vi "E816_All_VIs.vi"   [LabVIEW 2020]
doc: "This VI contains all high level and low level VIs valid for E-816. \nSee diagram for a survey of all E-816 high level and low level VIs. \nMenu / Browse / Show VI Hierarchy will show the file paths of the VIs. \nGlobal Variables are shown as Control as well as Indicator."
uses:
  Low Level/Communication.llb/Global1.vi
  Low Level/General command.llb/Controller names.ctl
  Low Level/Support.llb/Unbunde/bundle interface clusters for PI Terminal.vi
  Low Level/Communication.llb/Available DLL interfaces.ctl
  Low Level/Communication.llb/Available DLLs.ctl
  Low Level/Communication.llb/Available interfaces.ctl
  Low Level/Communication.llb/Termination character.ctl
  Low Level/General command.llb/Global2 (Array).vi
  Low Level/Communication.llb/Global DaisyChain.vi
  Low Level/Analog control.llb/Available Analog Commands.ctl
  Low Level/Analog control.llb/Global Analog.vi
panel:
  # "E-816 PI GCS LabVIEW driver set"
  # "This VI contains all high level and low level VIs valid for E-816. See diagram for a survey of all E-816 high \nlevel and low level VIs. Menu / Browse / Show VI Hierarchy will show the file paths of the VIs. Global \nVariables are shown as Control as well as Indicator."
types:
  T1 = typedef "Available Analog Commands.ctl" = enum16{"INITIALIZE", "VOL?", "VOL ", "CLOSE", "MOV", "POS?", "VCO", "VCO?", "WAIT_WF", "TMN?", "TMX?", "VEL", "VEL?", "SAI?", "MVR", "ERR?", "#24", "STP", "*IDN?", "#5", "STE", "DRR?", "W_Wave", "HLP?", "W/R_Wave"}
  T2 = typedef "Termination character.ctl" = enum16{"LF", "CR", "LFCR", "CRLF"}
  T3 = typedef "Available interfaces.ctl" = u16
  T4 = typedef "Available DLLs.ctl" = u16
  T5 = typedef "Available DLL interfaces.ctl" = u16
  T6 = typedef "Controller names.ctl" = enum16{"None", "Analog", "C-702", "C-843", "C-843.PM", "C-844", "C-848", "C-865", "C-866", "C-867", "C-880", "E-516", "E-517", "E-709", "E-710", "E-712", "E-725", "E-753", "E-755", "E-761", "E-816", "E-861", "F-206", "M-840", "M-850", "M-8X0", "Mercury", "Mercury_GCS"}
  T7 = cluster{"Conversion factor":dbl[], "Velocity":dbl[], "Velocity control mode":bool, "AO.Resolution":dbl, "Lower voltage limit (V)":dbl, "Upper voltage limit (V)":dbl, "AO_WF_T (s)":dbl, "AI Sample Rate":dbl, "AI Samples/Channel":i32, "Hyperbit":bool, "Offset (V)":dbl[], "Hyperbit StayOnPos":bool, "Gain (V)":dbl[], "Bit rate (Hz)":dbl, "PWM rate (Hz)":dbl, "HyperBit Password":string, "AO.MaxRate":dbl, "Conversion offset":dbl[]}[]
  T8 = cluster{"No. of devices":i32, "Port ID":i32, "Devices":string[], "Description":string}[]
  T9 = cluster{"Conn. axes":string[], "Controller name":T6}[]
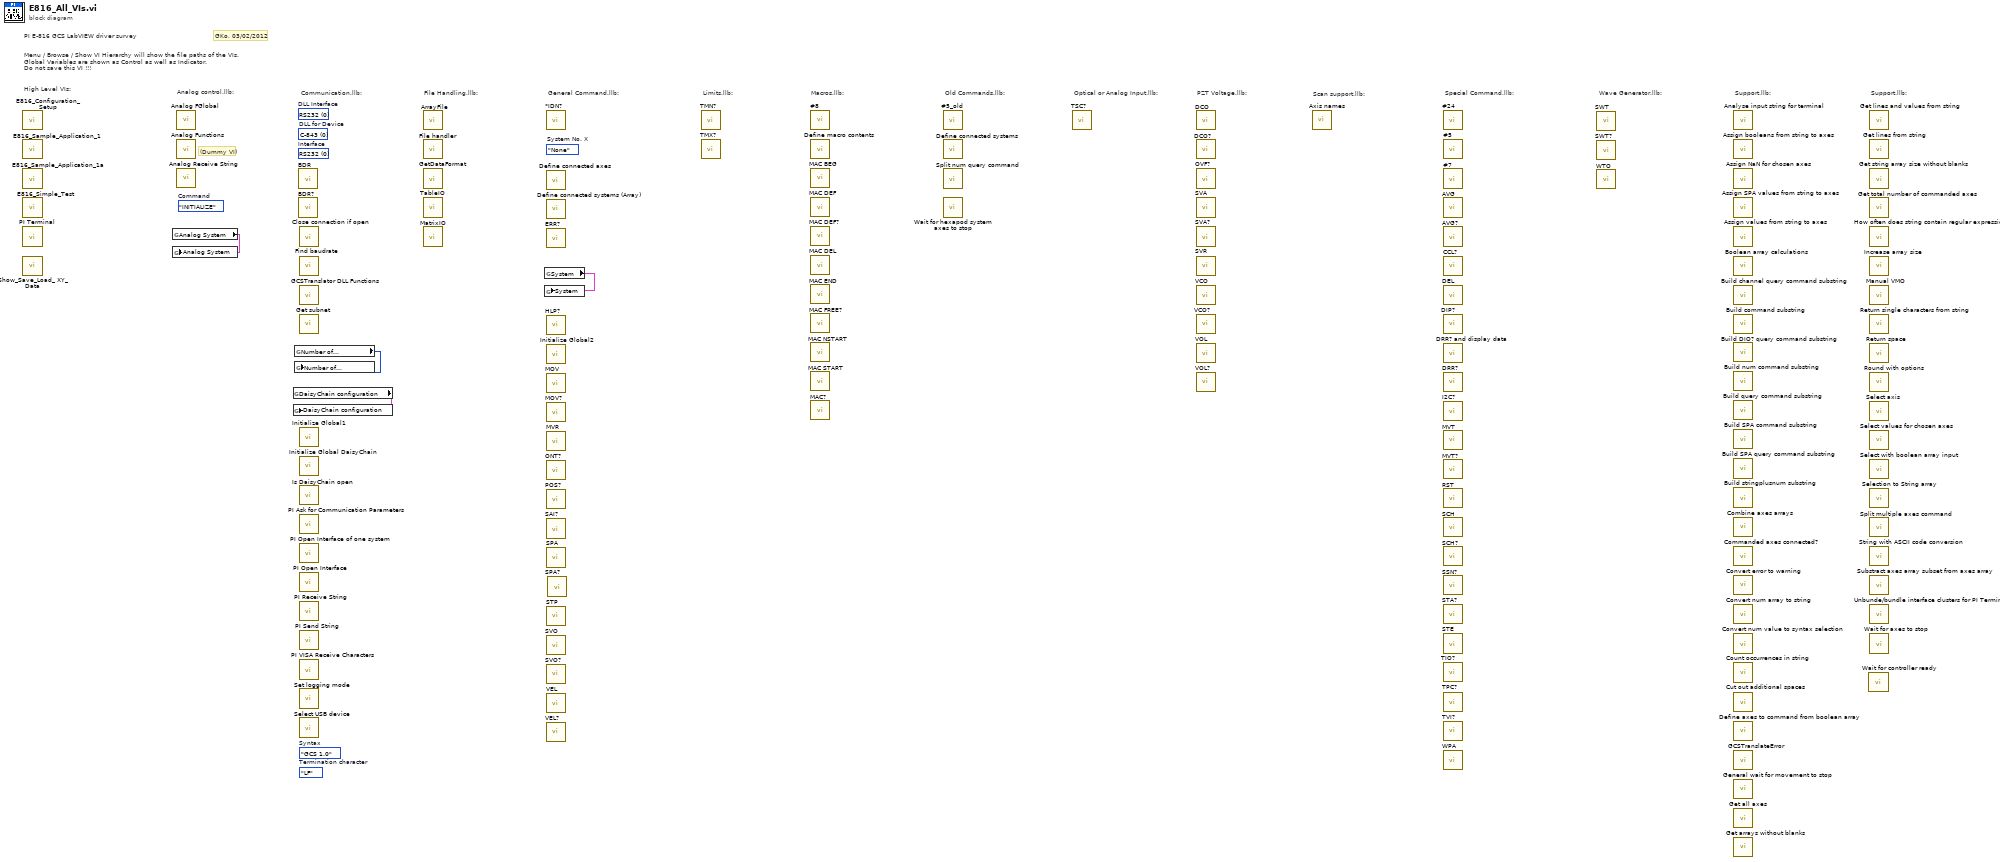
[diagram p0: block diagram]
diagram:
  (unwired) Available_Analog_Commands."INITIALIZE"  # Command
  (unwired) Termination_character."LF"  # Termination character
  (unwired) enum16{"GCS 1.0", "GCS 2.0"}."GCS 1.0"  # Syntax
  (unwired) T3 0 items=["RS232", "GPIB", "DLL", "TCP-IP"]  # Interface
  (unwired) T4 0 items=["C-843", "C-844", "E-710", "C-843.PM", "C-865", "E-761", "Mercury"]  # DLL for Device
  (unwired) T5 0 items=["RS232", "GPIB", "Board", "TCP-IP", "USB"]  # DLL Interface
  (unwired) Controller_names."None"  # System No. X
  # "Macros.llb:"
  # "Scan support.llb:"
  # "(Dummy VI)"
  # "GKo, 03/02/2012"
  # "High Level VIs:"
  # "Analog control.llb:"
  # "Support.llb:"
  # "Wave Generator.llb:"
  # "Support.llb:"
  # "Special Command.llb:"
  # "PZT Voltage.llb:"
  # "Optical or Analog Input.llb:"
  # "Old Commands.llb:"
  # "Limits.llb:"
  # "General Command.llb:"
  # "File Handling.llb:"
  # "Menu / Browse / Show VI Hierarchy will show the file paths of the VIs. \nGlobal Variables are shown as Control as well as Indicator.\nDo not save this VI !!!"
  # "PI E-816 GCS LabVIEW driver survey"
  # "Communication.llb:"
  n1 = call "E816_Configuration_Setup.vi"() -> ()  [unwired: 10 in, 10 out]
  n2 = call "E816_Sample_Application_1.vi"() -> ()  [unwired: 20 out]
  n3 = call "E816_Sample_Application_1a.vi"() -> ()  [unwired: 20 out]
  n4 = call "E816_Simple_Test.vi"() -> ()  [unwired: 20 out]
  n5 = call "PI Terminal.vi"() -> ()  [unwired: 20 out]
  n6 = call "Show_Save_Load_ XY_Data.vi"() -> ()  [unwired: 7 in, 13 out]
  n7 = global read "Global Analog.vi" "Analog System"() -> (w1:T7)
  n8 = global write "Global Analog.vi" "Analog System"(w1) -> ()
  n9 = call "Analog FGlobal.vi"() -> ()  [unwired: 3 in, 17 out]
  n10 = call "Analog Functions.vi"() -> ()  [unwired: 7 in, 13 out]
  n11 = call "Analog Receive String.vi"() -> ()  [unwired: 5 in, 15 out]
  n12 = global read "Global DaisyChain.vi" "DaisyChain configuration"() -> (w2:T8)
  n13 = global write "Global DaisyChain.vi" "DaisyChain configuration"(w2) -> ()
  n14 = global read "Global1.vi" "Number of\nsystems"() -> (w4:i32)
  n15 = global write "Global1.vi" "Number of\nsystems"(w4) -> ()
  n16 = call "BDR.vi"() -> ()  [unwired: 4 in, 16 out]
  n17 = call "BDR?.vi"() -> ()  [unwired: 2 in, 18 out]
  n18 = call "Close connection if open.vi"() -> ()  [unwired: 3 in, 17 out]
  n19 = call "Find baudrate.vi"() -> ()  [unwired: 10 in, 10 out]
  n20 = call "GCSTranslator DLL Functions.vi"() -> ()  [unwired: 7 in, 13 out]
  n21 = call "Get subnet.vi"() -> ()  [unwired: 20 out]
  n22 = call "Initialize Global1.vi"() -> ()  [unwired: 2 in, 18 out]
  n23 = call "Initialize Global DaisyChain.vi"() -> ()  [unwired: 2 in, 18 out]
  n24 = call "Is DaisyChain open.vi"() -> ()  [unwired: 2 in, 18 out]
  n25 = call "PI Ask for Communication Parameters.vi"() -> ()  [unwired: 20 out]
  n26 = call "PI Open Interface of one system.vi"() -> ()  [unwired: 12 in, 8 out]
  n27 = call "PI Open Interface.vi"() -> ()  [unwired: 12 in, 8 out]
  n28 = call "PI Receive String.vi"() -> ()  [unwired: 3 in, 17 out]
  n29 = call "PI Send String.vi"() -> ()  [unwired: 4 in, 16 out]
  n30 = call "PI VISA Receive Characters.vi"() -> ()  [unwired: 3 in, 17 out]
  n31 = call "Set logging mode.vi"() -> ()  [unwired: 4 in, 16 out]
  n32 = call "Select USB device.vi"() -> ()  [unwired: 5 in, 15 out]
  n33 = call "ArrayFile.vi"() -> ()  [unwired: 20 out]
  n34 = call "File handler.vi"() -> ()  [unwired: 6 in, 14 out]
  n35 = call "GetDataFormat.vi"() -> ()  [unwired: 2 in, 18 out]
  n36 = call "TableIO.vi"() -> ()  [unwired: 6 in, 14 out]
  n37 = call "MatrixIO.vi"() -> ()  [unwired: 7 in, 13 out]
  n38 = global read "Global2 (Array).vi" "System"() -> (w3:T9)
  n39 = global write "Global2 (Array).vi" "System"(w3) -> ()
  n40 = call "*IDN?.vi"() -> ()  [unwired: 2 in, 18 out]
  n41 = call "Define connected axes.vi"() -> ()  [unwired: 5 in, 15 out]
  n42 = call "Define connected systems (Array).vi"() -> ()  [unwired: 4 in, 16 out]
  n43 = call "ERR?.vi"() -> ()  [unwired: 2 in, 18 out]
  n44 = call "HLP?.vi"() -> ()  [unwired: 2 in, 18 out]
  n45 = call "Initialize Global2.vi"() -> ()  [unwired: 2 in, 18 out]
  n46 = call "MOV.vi"() -> ()  [unwired: 5 in, 15 out]
  n47 = call "MOV?.vi"() -> ()  [unwired: 5 in, 15 out]
  n48 = call "MVR.vi"() -> ()  [unwired: 5 in, 15 out]
  n49 = call "ONT?.vi"() -> ()  [unwired: 5 in, 15 out]
  n50 = call "POS?.vi"() -> ()  [unwired: 5 in, 15 out]
  n51 = call "SAI?.vi"() -> ()  [unwired: 5 in, 15 out]
  n52 = call "SPA.vi"() -> ()  [unwired: 10 in, 10 out]
  n53 = call "STP.vi"() -> ()  [unwired: 5 in, 15 out]
  n54 = call "SVO.vi"() -> ()  [unwired: 5 in, 15 out]
  n55 = call "SVO?.vi"() -> ()  [unwired: 5 in, 15 out]
  n56 = call "VEL.vi"() -> ()  [unwired: 6 in, 14 out]
  n57 = call "VEL?.vi"() -> ()  [unwired: 5 in, 15 out]
  n58 = call "SPA?.vi"() -> ()  [unwired: 7 in, 13 out]
  n59 = call "TMN?.vi"() -> ()  [unwired: 5 in, 15 out]
  n60 = call "TMX?.vi"() -> ()  [unwired: 5 in, 15 out]
  n61 = call "#8.vi"() -> ()  [unwired: 2 in, 18 out]
  n62 = call "Define macro contents.vi"() -> ()  [unwired: 3 in, 17 out]
  n63 = call "MAC BEG.vi"() -> ()  [unwired: 3 in, 17 out]
  n64 = call "MAC DEF.vi"() -> ()  [unwired: 3 in, 17 out]
  n65 = call "MAC DEF?.vi"() -> ()  [unwired: 2 in, 18 out]
  n66 = call "MAC DEL.vi"() -> ()  [unwired: 4 in, 16 out]
  n67 = call "MAC END.vi"() -> ()  [unwired: 2 in, 18 out]
  n68 = call "MAC FREE?.vi"() -> ()  [unwired: 2 in, 18 out]
  n69 = call "MAC NSTART.vi"() -> ()  [unwired: 5 in, 15 out]
  n70 = call "MAC START.vi"() -> ()  [unwired: 4 in, 16 out]
  n71 = call "MAC?.vi"() -> ()  [unwired: 4 in, 16 out]
  n72 = call "#5_old.vi"() -> ()  [unwired: 2 in, 18 out]
  n73 = call "Define connected systems.vi"() -> ()  [unwired: 4 in, 16 out]
  n74 = call "Split num query command.vi"() -> ()  [unwired: 4 in, 16 out]
  n75 = call "Wait for hexapod system axes to stop.vi"() -> ()  [unwired: 5 in, 15 out]
  n76 = call "TSC?.vi"() -> ()  [unwired: 2 in, 18 out]
  n77 = call "DCO.vi"() -> ()  [unwired: 4 in, 16 out]
  n78 = call "DCO?.vi"() -> ()  [unwired: 5 in, 15 out]
  n79 = call "OVF?.vi"() -> ()  [unwired: 5 in, 15 out]
  n80 = call "SVA.vi"() -> ()  [unwired: 5 in, 15 out]
  n81 = call "SVA?.vi"() -> ()  [unwired: 5 in, 15 out]
  n82 = call "SVR.vi"() -> ()  [unwired: 5 in, 15 out]
  n83 = call "VCO.vi"() -> ()  [unwired: 4 in, 16 out]
  n84 = call "VCO?.vi"() -> ()  [unwired: 5 in, 15 out]
  n85 = call "VOL.vi"() -> ()  [unwired: 5 in, 15 out]
  n86 = call "VOL?.vi"() -> ()  [unwired: 5 in, 15 out]
  n87 = call "Axis names.vi"() -> ()  [unwired: 1 in, 19 out]
  n88 = call "#24.vi"() -> ()  [unwired: 2 in, 18 out]
  n89 = call "#5.vi"() -> ()  [unwired: 2 in, 18 out]
  n90 = call "#7.vi"() -> ()  [unwired: 2 in, 18 out]
  n91 = call "AVG.vi"() -> ()  [unwired: 3 in, 17 out]
  n92 = call "AVG?.vi"() -> ()  [unwired: 2 in, 18 out]
  n93 = call "CCL?.vi"() -> ()  [unwired: 2 in, 18 out]
  n94 = call "DEL.vi"() -> ()  [unwired: 3 in, 17 out]
  n95 = call "DIP?.vi"() -> ()  [unwired: 5 in, 15 out]
  n96 = call "DRR? and display data.vi"() -> ()  [unwired: 7 in, 13 out]
  n97 = call "DRR?.vi"() -> ()  [unwired: 7 in, 13 out]
  n98 = call "I2C?.vi"() -> ()  [unwired: 2 in, 18 out]
  n99 = call "MVT.vi"() -> ()  [unwired: 5 in, 15 out]
  n100 = call "MVT?.vi"() -> ()  [unwired: 5 in, 15 out]
  n101 = call "RST.vi"() -> ()  [unwired: 5 in, 15 out]
  n102 = call "SCH.vi"() -> ()  [unwired: 3 in, 17 out]
  n103 = call "SCH?.vi"() -> ()  [unwired: 2 in, 18 out]
  n104 = call "SSN?.vi"() -> ()  [unwired: 4 in, 16 out]
  n105 = call "STA?.vi"() -> ()  [unwired: 5 in, 15 out]
  n106 = call "STE.vi"() -> ()  [unwired: 6 in, 14 out]
  n107 = call "TIO?.vi"() -> ()  [unwired: 2 in, 18 out]
  n108 = call "TPC?.vi"() -> ()  [unwired: 2 in, 18 out]
  n109 = call "TVI?.vi"() -> ()  [unwired: 3 in, 17 out]
  n110 = call "WPA.vi"() -> ()  [unwired: 7 in, 13 out]
  n111 = call "SWT.vi"() -> ()  [unwired: 6 in, 14 out]
  n112 = call "SWT?.vi"() -> ()  [unwired: 4 in, 16 out]
  n113 = call "WTO.vi"() -> ()  [unwired: 6 in, 14 out]
  n114 = call "Analyse input string for terminal.vi"() -> ()  [unwired: 2 in, 18 out]
  n115 = call "Assign booleans from string to axes.vi"() -> ()  [unwired: 5 in, 15 out]
  n116 = call "Assign NaN for chosen axes.vi"() -> ()  [unwired: 4 in, 16 out]
  n117 = call "Assign SPA values from string to axes.vi"() -> ()  [unwired: 7 in, 13 out]
  n118 = call "Assign values from string to axes.vi"() -> ()  [unwired: 6 in, 14 out]
  n119 = call "Boolean array calculations.vi"() -> ()  [unwired: 4 in, 16 out]
  n120 = call "Build channel query command substring.vi"() -> ()  [unwired: 7 in, 13 out]
  n121 = call "Build command substring.vi"() -> ()  [unwired: 7 in, 13 out]
  n122 = call "Build DIO? query command substring.vi"() -> ()  [unwired: 6 in, 14 out]
  n123 = call "Build num command substring.vi"() -> ()  [unwired: 3 in, 17 out]
  n124 = call "Build query command substring.vi"() -> ()  [unwired: 5 in, 15 out]
  n125 = call "Build SPA command substring.vi"() -> ()  [unwired: 10 in, 10 out]
  n126 = call "Build SPA query command substring.vi"() -> ()  [unwired: 5 in, 15 out]
  n127 = call "Build stringplusnum substring.vi"() -> ()  [unwired: 10 in, 10 out]
  n128 = call "Combine axes arrays.vi"() -> ()  [unwired: 2 in, 18 out]
  n129 = call "Commanded axes connected?.vi"() -> ()  [unwired: 3 in, 17 out]
  n130 = call "Convert error to warning.vi"() -> ()  [unwired: 2 in, 18 out]
  n131 = call "Convert num array to string.vi"() -> ()  [unwired: 2 in, 18 out]
  n132 = call "Convert num value to syntax selection.vi"() -> ()  [unwired: 1 in, 19 out]
  n133 = call "Count occurrences in string.vi"() -> ()  [unwired: 2 in, 18 out]
  n134 = call "Cut out additional spaces.vi"() -> ()  [unwired: 2 in, 18 out]
  n135 = call "Define axes to command from boolean array.vi"() -> ()  [unwired: 4 in, 16 out]
  n136 = call "GCSTranslateError.vi"() -> ()  [unwired: 1 in, 19 out]
  n137 = call "General wait for movement to stop.vi"() -> ()  [unwired: 8 in, 12 out]
  n138 = call "Get all axes.vi"() -> ()  [unwired: 1 in, 19 out]
  n139 = call "Get arrays without blanks.vi"() -> ()  [unwired: 3 in, 17 out]
  n140 = call "Wait for controller ready.vi"() -> ()  [unwired: 4 in, 16 out]
  n141 = call "Get lines and values from string.vi"() -> ()  [unwired: 2 in, 18 out]
  n142 = call "Get lines from string.vi"() -> ()  [unwired: 3 in, 17 out]
  n143 = call "Get string array size without blanks.vi"() -> ()  [unwired: 1 in, 19 out]
  n144 = call "Get total number of commanded axes.vi"() -> ()  [unwired: 2 in, 18 out]
  n145 = call "How often does string contain regular expression?.vi"() -> ()  [unwired: 2 in, 18 out]
  n146 = call "Increase array size.vi"() -> ()  [unwired: 3 in, 17 out]
  n147 = call "Manual VMO.vi"() -> ()  [unwired: 6 in, 14 out]
  n148 = call "Return single characters from string.vi"() -> ()  [unwired: 3 in, 17 out]
  n149 = call "Return space.vi"() -> ()  [unwired: 2 in, 18 out]
  n150 = call "Round with options.vi"() -> ()  [unwired: 4 in, 16 out]
  n151 = call "Select axis.vi"() -> ()  [unwired: 2 in, 18 out]
  n152 = call "Select values for chosen axes.vi"() -> ()  [unwired: 5 in, 15 out]
  n153 = call "Select with boolean array input.vi"() -> ()  [unwired: 4 in, 16 out]
  n154 = call "Selection to String array.vi"() -> ()  [unwired: 2 in, 18 out]
  n155 = call "Split multiple axes command.vi"() -> ()  [unwired: 9 in, 11 out]
  n156 = call "String with ASCII code conversion.vi"() -> ()  [unwired: 1 in, 19 out]
  n157 = call "Substract axes array subset from axes array.vi"() -> ()  [unwired: 2 in, 18 out]
  n158 = call "Unbunde/bundle interface clusters for PI Terminal.vi"() -> ()  [unwired: 6 in, 14 out]
  n159 = call "Wait for axes to stop.vi"() -> ()  [unwired: 7 in, 13 out]
